vi "Instrument Manager Loop.vi"(8 "System Control":refnum<queue>, 11 "Instrument Manager":refnum<queue>) -> (0 "error out":errorcluster)   [LabVIEW 2020, in "Waters Patrol UPLC Report Parser.lvlib" / "Instrument Manager.lvlib"]
uses:
  Instrument Manager/Instrument Manager.lvlib
  support/Message Queue/Message Cluster.ctl
  Instrument Manager/Instrument State.ctl
  <vilib>/Utility/error.llb/Error Cluster From Error Code.vi
  <vilib>/ErrorRing/Error Ring.xnode
  support/Message Queue/Message Queue.lvlib
  Waters Patrol UPLC Report Parser.lvlib
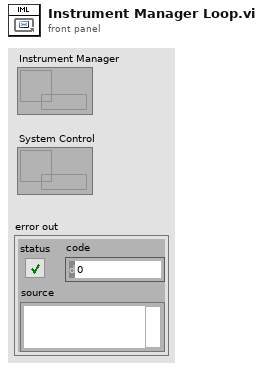
[diagram p1: front panel]
types:
  T1 = cluster{"Time Stamp":timestamp, "Peaks":string[][]}[]
  T2 = typedef "Waters Patrol UPLC Report Parser.lvlib/Instrument Manager.lvlib/Instrument State.ctl" = cluster{"Data Directory":path, "Last Report Number":i32, "Yield":dbl, "Max Concentration (mM)":dbl, "Report File Pattern":string, "Current Data File":path, "Peak Data Array":cluster{"Time Stamp":timestamp, "Peaks":string[][]}[], "Average Peak Data":cluster{"Time Stamp":timestamp, "Peaks":string[][]}, "Points to Average":i32}
  T3 = cluster{"seconds since 1Jan1904":timestamp, "Peaks":string[][]}
  T4 = cluster{"seconds since 1Jan1904":timestamp, "Peaks":string[][]}[]
  T5 = cluster{"Time Stamp":timestamp, "Peaks":string[][]}
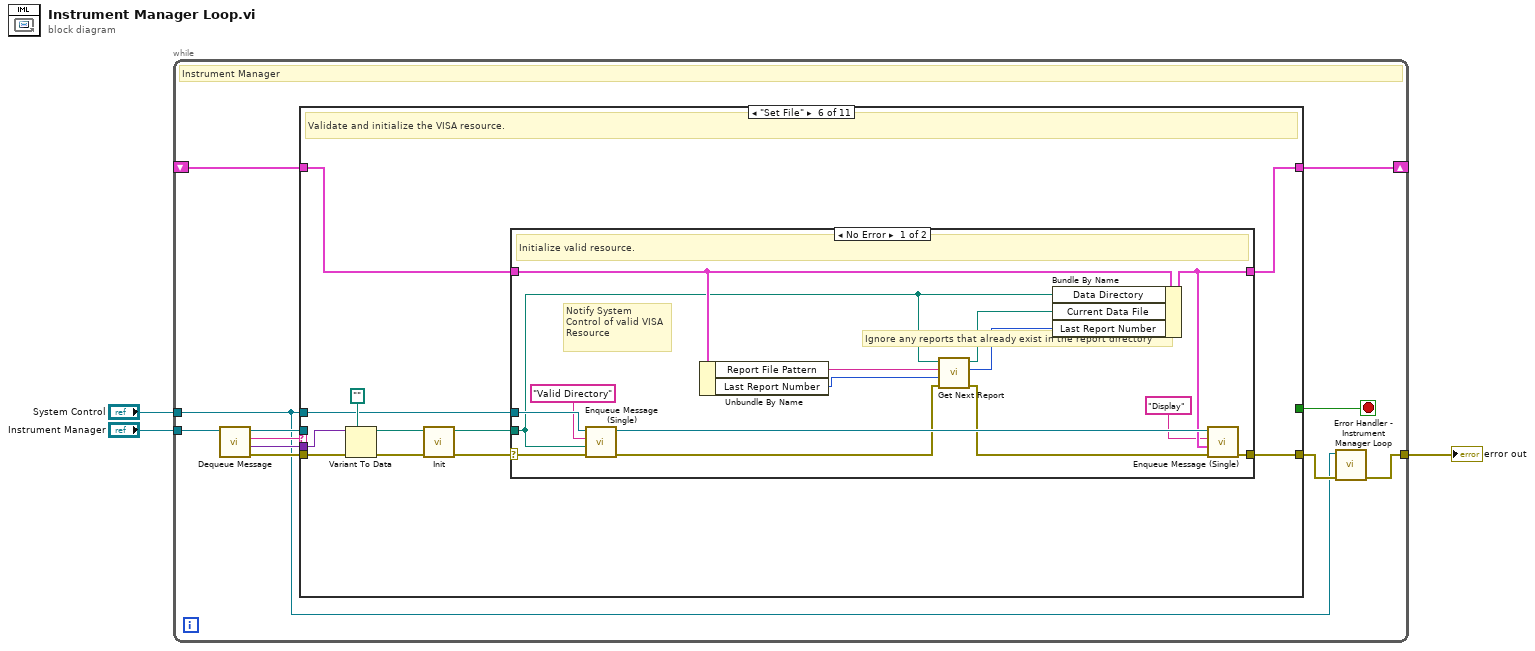
[diagram p0: block diagram]
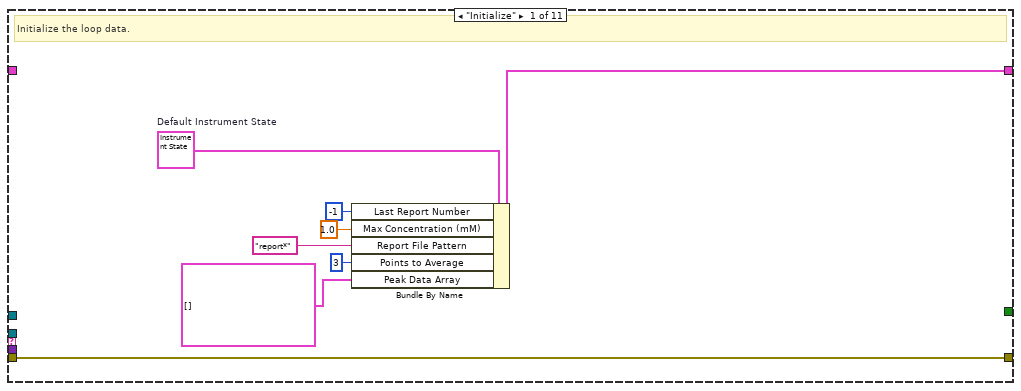
[diagram p2: hidden frame]
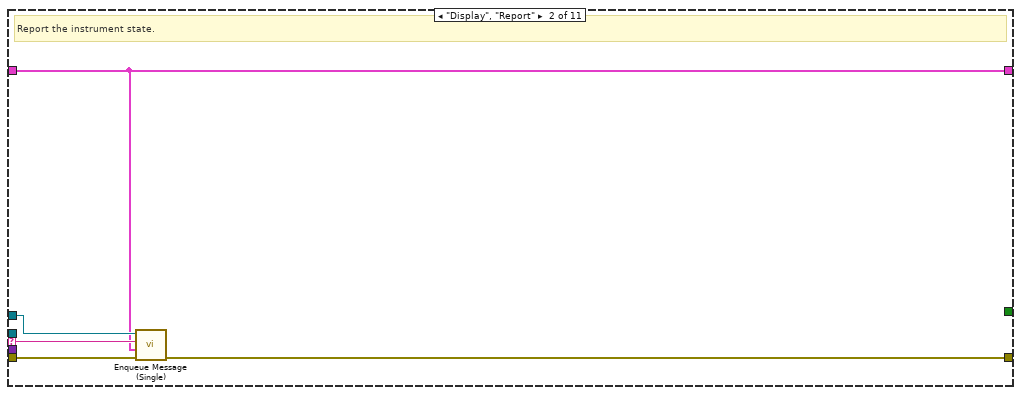
[diagram p3: hidden frame]
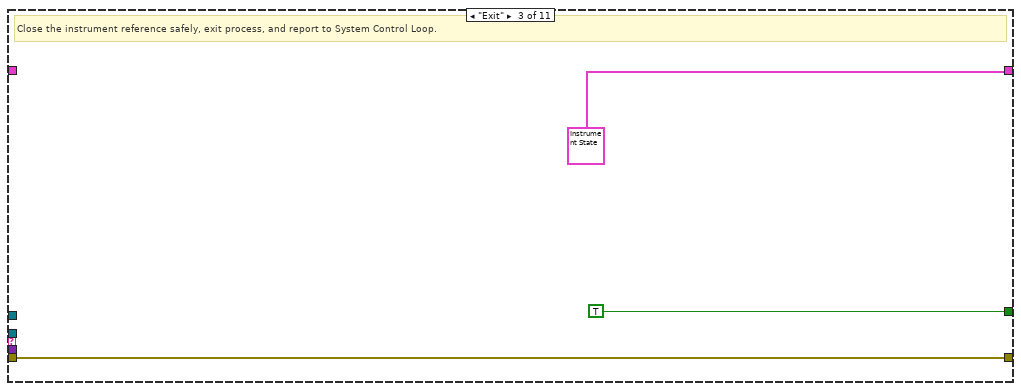
[diagram p4: hidden frame]
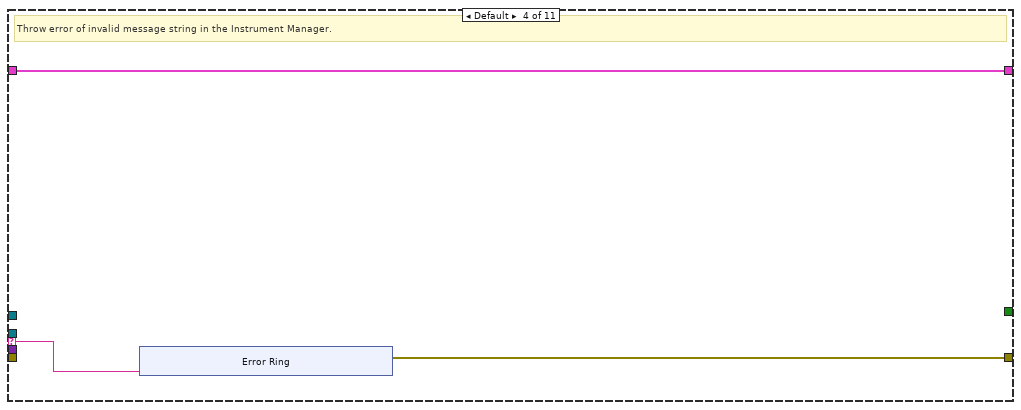
[diagram p5: hidden frame]
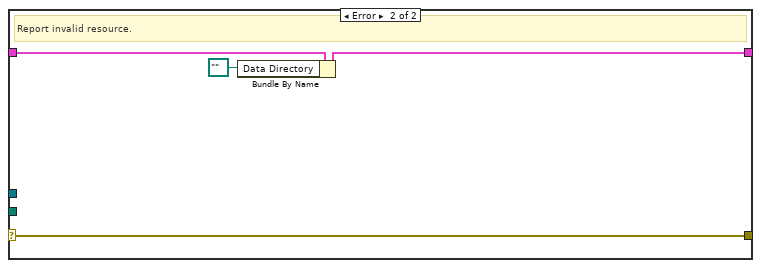
[diagram p7: hidden frame]
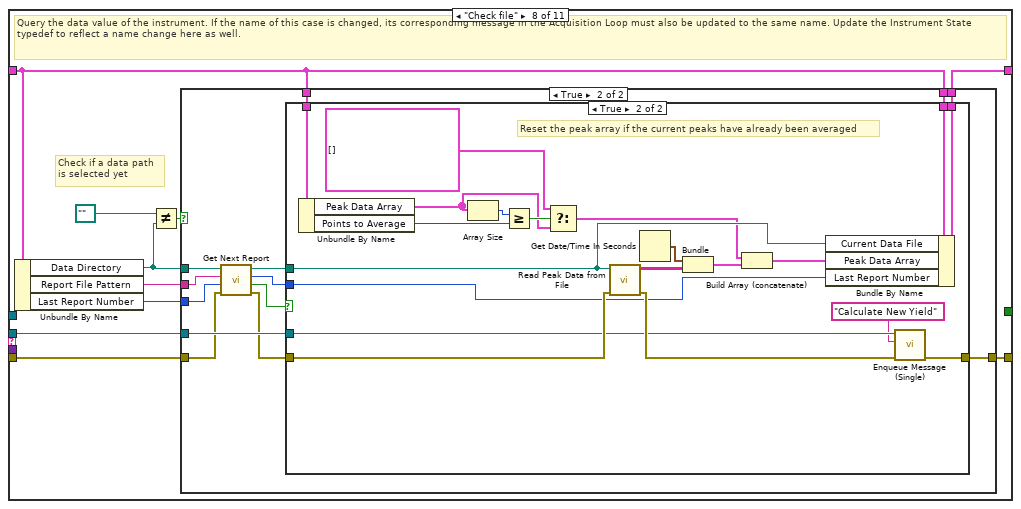
[diagram p9: hidden frame]
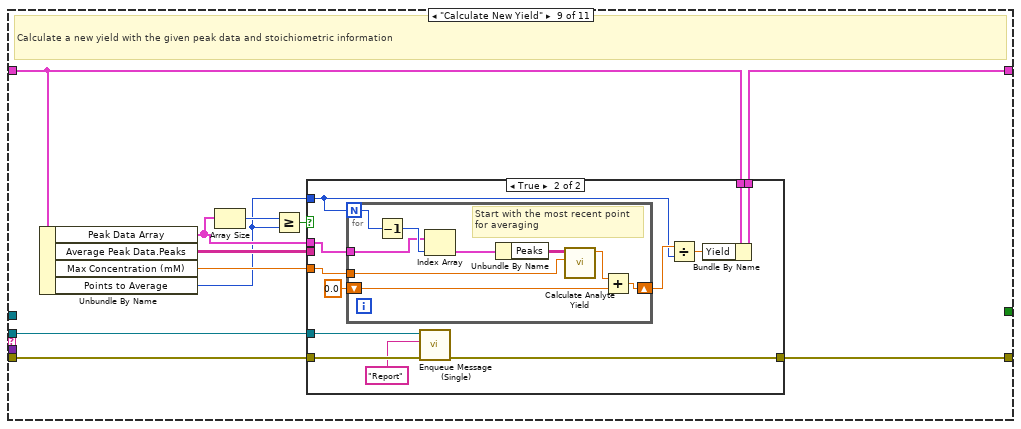
[diagram p12: hidden frame]
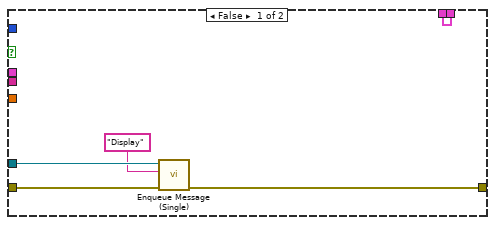
[diagram p13: hidden frame]
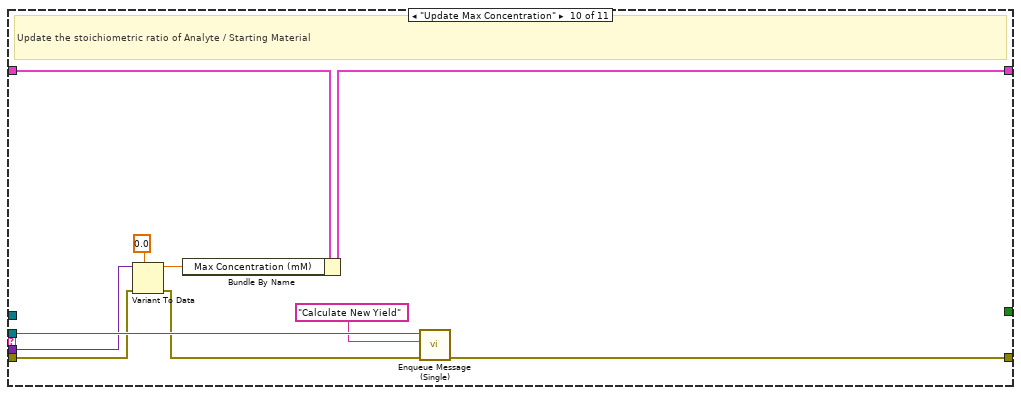
[diagram p14: hidden frame]
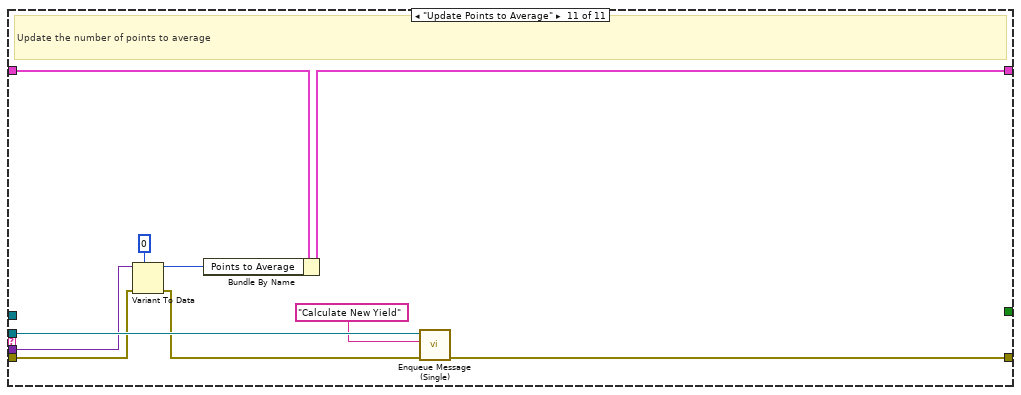
[diagram p15: hidden frame]
diagram:
  n1 = while {
    tunnel: "Instrument Manager" -> [w14]
    tunnel: "System Control" -> [w4]
    tunnel: [w8] -> w1
    shift-right: [w6] -> _
    shift-left: _ -> [w7]
    stop <- w5 stop-if-true
    # "Instrument Manager"
    n2 = call "Dequeue Message.vi"("Message Queue"=w14) -> ("error out"=w10:errorcluster, "Message Data"=w11:variant, "Message"=w13:string, "dup Message Queue"=w12:refnum<queue>)  [unwired: 7 in]
    n3 = case shown="\"Set File\"" w13 {
      selector: w13 -> [_ w25 _ w32 _ _ _ _ _ _ _]
      tunnel: w12 -> [_ _ _ _ _ _ _ w78 w128 w165 w175]
      tunnel: w4 -> [_ w26 _ _ _ w43 _ _ _ _ _]
      tunnel: w11 -> [_ _ _ _ _ w50 _ _ _ w161 w171]
      tunnel: w10 -> [w21 w27 w28 _ w41 w49 w74 w83 w130 w163 w173]
      tunnel: [w21 w23 w28 w31 w41 w53 w74 w79 w129 w166 w176] -> w9
      tunnel: w7 -> [_ w24 _ w33 w42 w52 w73 w76 w131 w167 w177]
      tunnel: [w20 w24 T2 {"Data Directory"=path "", "Last Report Number"=0, "Yield"=0.0, "Max Concentration (mM)"=1.0, "Report File Pattern"="", "Current Data File"=path "", "Peak Data Array"=[], "Average Peak Data"={"Time Stamp"=timestamp(0 s since 1904-01-01), "Peaks"=[]}, "Points to Average"=3} w33 w42 w51 w73 w84 w132 w168 w178] -> w6
      tunnel: [_ _ TRUE _ _ _ _ _ _ _ _] -> w5
      frame "Initialize" {
        w22 = T2 {"Data Directory"=path "", "Last Report Number"=0, "Yield"=0.0, "Max Concentration (mM)"=1.0, "Report File Pattern"="", "Current Data File"=path "", "Peak Data Array"=[], "Average Peak Data"={"Time Stamp"=timestamp(0 s since 1904-01-01), "Peaks"=[]}, "Points to Average"=3}  # Default Instrument State
        # "Initialize the loop data."
        n4 = Bundle By Name(cluster=w22, "Last Report Number"=-1, "Max Concentration (mM)"=1.0 ("Stoichiometry"), "Report File Pattern"="report*", "Points to Average"=3, "Peak Data Array"=T1 []) -> (w20:T2)
      }
      frame "Display", "Report" {
        # "Report the instrument state."
        n5 = call "Enqueue Message (Single).vi"("error in (no error)"=w27, "Message Data"=w24, "Message"=w25, "Message Queue"=w26) -> ("error out"=w23:errorcluster)  [unwired: 6 in, 1 out]
      }
      frame "Exit" {
        # "Close the instrument reference safely, exit process, and report to System Control Loop."
      }
      frame Default {
        # "Throw error of invalid message string in the Instrument Manager."
        n6 = xnode "Error Ring"("parameter 0"=w32) -> ("error out"=w31:errorcluster)
      }
      frame "--- Copy This Frame ---" {
        # "Copy this frame and add responses to instrument specific messages."
      }
      frame "Set File" {
        # "Validate and initialize the VISA resource."
        n7 = Variant To Data(error in=w49, type=path "", Variant=w50) -> (data=w47:path, error out=w48:errorcluster)
        n8 = call "Init.vi"("error in (no error)"=w48, "VISA resource in"=w47) -> ("error out"=w44:errorcluster, "Data Output File Out"=w45:path)  [unwired: 8 in]
        n9 = case shown="No Error" w44 {
          selector: w44 -> [w68 w70]
          tunnel: w45 -> [w64 _]
          tunnel: [w56 w70] -> w53
          tunnel: w52 -> [w65 w72]
          tunnel: [w55 w71] -> w51
          tunnel: w43 -> [w67 _]
          frame No Error {
            # "Ignore any reports that already exist in the report directory"
            # "Notify System Control of valid VISA Resource"
            # "Initialize valid resource."
            n10 = call "Enqueue Message (Single).vi"("error in (no error)"=w68, "Message Data"=w64, "Message"="Valid Directory", "Message Queue"=w67) -> ("error out"=w59:errorcluster, "dup Message Queue"=w60:refnum<queue>)  [unwired: 6 in]
            n11 = Unbundle By Name(w65) -> ("Report File Pattern"=w63:string, "Last Report Number"=w62:i32)
            n12 = call "Get Next Report.vi"("error in"=w59, "Last Report Number (-1)"=w62, "Report File Pattern"=w63, "Data Directory"=w64) -> ("error out"=w57:errorcluster, "Report number"=w61:i32, "Report Path"=w58:path)  [unwired: 4 in, 1 out]
            n13 = Bundle By Name(cluster=w65, "Data Directory"=w64, "Current Data File"=w58, "Last Report Number"=w61) -> (w55:T2)
            n14 = call "Enqueue Message (Single).vi"("error in (no error)"=w57, "Message Data"=w55, "Message"="Display", "Message Queue"=w60) -> ("error out"=w56:errorcluster)  [unwired: 6 in, 1 out]
          }
          frame Error {
            # "Report invalid resource."
            n15 = Bundle By Name(cluster=w72, "Data Directory"=path "" ("Data File")) -> (w71:T2)
          }
        }
      }
      frame "--- Copy for Get State Messages ---" {
        # "#CodeNeeded - Use the Bundle by Name function to bundle the new state value into the Instrument State cluster."
        # "#CodeNeeded - Add instrument driver call to query the instrument state requested"
        # "Duplicate this case for messages cases that will query the instrument state."
      }
      frame "Check file" {
        # "Check if a data path\nis selected yet"
        # "Query the data value of the instrument. If the name of this case is changed, its corresponding message in the Acquisition Loop must also be updated to the same name. Update the Instrument State typedef to reflect a name change here as well."
        n16 = Unbundle By Name(w76) -> ("Data Directory"=w82:path, "Report File Pattern"=w77:string, "Last Report Number"=w75:i32)
        n17 = Not Equal?(x=path "", y=w82) -> (x != y?=w80:bool)
        n18 = case shown="True" w80 {
          tunnel: [w85 w96] -> w84
          tunnel: w82 -> [_ w92]
          tunnel: w83 -> [w86 w88]
          tunnel: w77 -> [_ w90]
          tunnel: [w86 w99] -> w79
          tunnel: w78 -> [_ w98]
          tunnel: w76 -> [w85 w97]
          tunnel: w76 -> [_ w91]
          tunnel: w75 -> [_ w89]
          frame False {
            # "Do nothing if no directory is selected"
          }
          frame True {
            n19 = call "Get Next Report.vi"("error in"=w88, "Last Report Number (-1)"=w89, "Report File Pattern"=w90, "Data Directory"=w92) -> ("error out"=w87:errorcluster, "New report?"=w95:bool, "Report number"=w93:i32, "Report Path"=w94:path)  [unwired: 4 in]
            n20 = case shown="True" w95 {
              tunnel: w94 -> [_ w111]
              tunnel: w87 -> [w101 w121]
              tunnel: [w101 w119] -> w99
              tunnel: w98 -> [_ w118]
              tunnel: w97 -> [w100 w114]
              tunnel: [w100 w113] -> w96
              tunnel: w93 -> [_ w112]
              tunnel: w91 -> [_ w109]
              frame False {
              }
              frame True {
                # "Reset the peak array if the current peaks have already been averaged"
                n21 = Unbundle By Name(w109) -> ("Peak Data Array"=w105:T1, "Points to Average"=w102:i32)
                n22 = Array Size(array=w105) -> (size(s)=w107:i32)
                n23 = Greater Or Equal?(x=w107, y=w102) -> (x >= y?=w106:bool)
                n24 = Select(t=T1 [] ("Peak Data Array"), s=w106, f=w105) -> (s? t:f=w103:T1)
                n25 = call "Read Peak Data from File.vi"("error in (no error)"=w121, "Data File"=w111) -> ("error out"=w120:errorcluster, "Peaks"=w115:string[][])  [unwired: 8 in]
                n26 = Get Date/Time In Seconds() -> (seconds since 1Jan1904=w116:timestamp)
                n27 = Bundle("seconds since 1Jan1904"=w116, "Peaks"=w115) -> (w110:T3)  [unwired: 1 in]
                n28 = Build Array (concatenate)(w103, w110) -> (w108:T4)
                n29 = Bundle By Name(cluster=w114, "Current Data File"=w111, "Peak Data Array"=w108, "Last Report Number"=w112) -> (w113:T2)
                n30 = call "Enqueue Message (Single).vi"("error in (no error)"=w120, "Message"="Calculate New Yield", "Message Queue"=w118) -> ("error out"=w119:errorcluster)  [unwired: 7 in, 1 out]
              }
            }
          }
        }
      }
      frame "Calculate New Yield" {
        # "Calculate a new yield with the given peak data and stoichiometric information"
        n31 = Unbundle By Name(w131) -> ("Peak Data Array"=w124:T1, "Average Peak Data.Peaks"=w125:string[][], "Max Concentration (mM)"=w127:dbl, "Points to Average"=w122:i32)
        n32 = Array Size(array=w124) -> (size(s)=w123:i32)
        n33 = Greater Or Equal?(x=w123, y=w122) -> (x >= y?=w126:bool)
        n34 = case shown="True" w126 {
          tunnel: [w137 w149] -> w132
          tunnel: w131 -> [w137 w148]
          tunnel: w130 -> [w136 w147]
          tunnel: [w135 w138] -> w129
          tunnel: w128 -> [w134 w146]
          tunnel: w127 -> [_ w144]
          tunnel: w125 -> [_ _]
          tunnel: w124 -> [_ w143]
          tunnel: w122 -> [_ w139]
          frame False {
            n35 = call "Enqueue Message (Single).vi"("error in (no error)"=w136, "Message"="Display", "Message Queue"=w134) -> ("error out"=w135:errorcluster)  [unwired: 7 in, 1 out]
          }
          frame True {
            n36 = for {
              N: w139 -> [w153]
              tunnel: w144 -> [w158]
              tunnel: w143 -> [w151]
              shift-right: [w154] -> w141
              shift-left: 0.0 -> [w156]
              # "Start with the most recent point\nfor averaging"
              n37 = Decrement(x=w153) -> (x-1=w152:i32)
              n38 = Index Array(array=w151, index=w152) -> (element=w150:T5)
              n39 = Unbundle By Name(w150) -> ("Peaks"=w157:string[][])
              n40 = call "Calculate Analyte Yield.vi"("Max Concentration"=w158, "Peaks"=w157) -> ("Yield out"=w155:dbl)  [unwired: 9 in]
              n41 = Add(x=w155, y=w156) -> (x+y=w154:dbl)
            }
            n42 = call "Enqueue Message (Single).vi"("error in (no error)"=w147, "Message"="Report", "Message Queue"=w146) -> ("error out"=w138:errorcluster)  [unwired: 7 in, 1 out]
            n43 = Divide(x=w141, y=w139) -> (x/y=w140:dbl)
            n44 = Bundle By Name(cluster=w148, "Yield"=w140) -> (w149:T2)
          }
        }
      }
      frame "Update Max Concentration" {
        # "Update the stoichiometric ratio of Analyte / Starting Material"
        n45 = Variant To Data(error in=w163, type=0.0, Variant=w161) -> (data=w159:dbl, error out=w162:errorcluster)
        n46 = Bundle By Name(cluster=w167, "Max Concentration (mM)"=w159) -> (w168:T2)
        n47 = call "Enqueue Message (Single).vi"("error in (no error)"=w162, "Message"="Calculate New Yield", "Message Queue"=w165) -> ("error out"=w166:errorcluster)  [unwired: 7 in, 1 out]
      }
      frame "Update Points to Average" {
        # "Update the number of points to average"
        n48 = Variant To Data(error in=w173, type=0, Variant=w171) -> (data=w169:i32, error out=w172:errorcluster)
        n49 = Bundle By Name(cluster=w177, "Points to Average"=w169) -> (w178:T2)
        n50 = call "Enqueue Message (Single).vi"("error in (no error)"=w172, "Message"="Calculate New Yield", "Message Queue"=w175) -> ("error out"=w176:errorcluster)  [unwired: 7 in, 1 out]
      }
    }
    n51 = call "Error Handler - Instrument Manager Loop.vi"("error in (no error)"=w9, "Message Queue"=w4) -> ("dup error in"=w8:errorcluster)  [unwired: 8 in, 1 out]
  }
  "error out" <- w1
